vi "zad4.vi"() -> ()   [LabVIEW 2023]
panel:
  in  "?":bool
  in  "User":string
  in  "?":bool
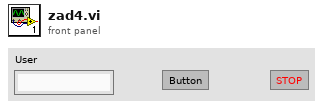
[diagram p1: front panel]
types:
  T1 = enum16{"open", "replace", "create", "open or create", "replace or create", "replace or create with confirmation"}
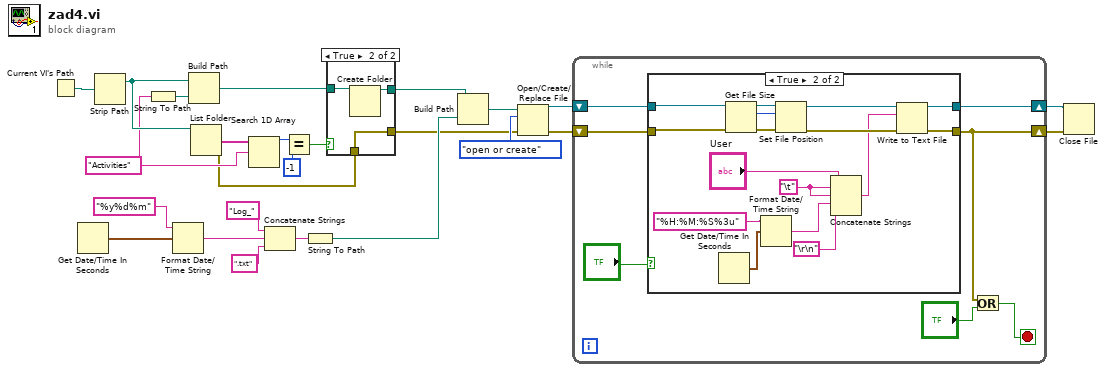
[diagram p0: block diagram]
diagram:
  w12 = "Activities" ("element")
  n1 = Current VI's Path() -> (path=w25:path)
  n2 = Get Date/Time In Seconds() -> (seconds since 1Jan1904=w22:timestamp)
  n3 = Strip Path(path=w25) -> (stripped path=w15:path)  [unwired: 1 out]
  n4 = String To Path(string=w12) -> (path=w13:path)
  n5 = Format Date/Time String(time format string (%c)="%y%d%m", seconds (now)=w22) -> (date/time string=w20:string)  [unwired: 1 in]
  n6 = Build Path(base path=w15, name or relative path=w13) -> (appended path=w7:path)
  n7 = List Folder(path=w15) -> (folder names=w14:string[], error out=w8:errorcluster)  [unwired: 3 in, 2 out]
  n8 = Search 1D Array(1D array=w14, element=w12) -> (index of element=w11:i32)  [unwired: 1 in]
  n9 = Concatenate Strings("Log_" ("string"), w20, ".txt" ("string")) -> (w17:string)
  n10 = Equal?(x=w11, y=-1) -> (x = y?=w9:bool)
  n11 = String To Path(string=w17) -> (path=w16:path)
  n12 = case shown="True" w9 {
    tunnel: [w26 w30] -> w5
    tunnel: w8 -> [w26 w30]
    tunnel: w7 -> [w27 w29]
    tunnel: [w27 w28] -> w6
    frame False {
    }
    frame True {
      n13 = Create Folder(path (use dialog)=w29) -> (created path=w28:path)  [unwired: 2 in, 2 out]
    }
  }
  n14 = Build Path(base path=w6, name or relative path=w16) -> (appended path=w23:path)
  n15 = Open/Create/Replace File(file path (use dialog)=w23, error in=w5, operation (0:open)=T1."open or create") -> (refnum out=w2:refnum<file>, error out=w4:errorcluster)  [unwired: 3 in, 1 out]
  n16 = while {
    shift-right: [w34] -> w1
    shift-left: w2 -> [w35]
    shift-right: [w32] -> w3
    shift-left: w4 -> [w36]
    stop <- w31 stop-if-true
    n17 = case shown="True" "?" {
      tunnel: w36 -> [w39 w51]
      tunnel: [w39 w47] -> w32
      tunnel: w35 -> [w38 w52]
      tunnel: [w38 w50] -> w34
      frame False {
      }
      frame True {
        w44 = "\t"
        n18 = Get Date/Time In Seconds() -> (seconds since 1Jan1904=w42:timestamp)
        n19 = Get File Size(file=w52, error in=w51) -> (refnum out=w53:refnum<file>, size (in bytes)=w54:i64, 0:w55:errorcluster)
        n20 = Format Date/Time String(time format string (%c)="%H:%M:%S%3u", seconds (now)=w42) -> (date/time string=w40:string)  [unwired: 1 in]
        n21 = Set File Position(offset (in bytes) (0)=w54, refnum=w53, error in=w55) -> (refnum out=w49:refnum<file>, error out=w48:errorcluster)  [unwired: 1 in]
        n22 = Concatenate Strings("User", w44, w44, w40, "\r\n") -> (w46:string)
        n23 = Write to Text File(file (use dialog)=w49, text=w46, error in=w48) -> (refnum out=w50:refnum<file>, error out=w47:errorcluster)  [unwired: 1 in, 1 out]
      }
    }
    n24 = Or(x=w32, y="?") -> (x .or. y?=w31:bool)
  }
  n25 = Close File(refnum=w1, error in=w3) -> ()  [unwired: 2 out]
